vi "waveform_array_to_xy_array.vi"(1 "waveform array":waveform(dbl)[](array[waveform])) -> (0 "XY array":cluster{timestamp[], "Y":dbl[]}[](array[cluster]))   [LabVIEW 2019]
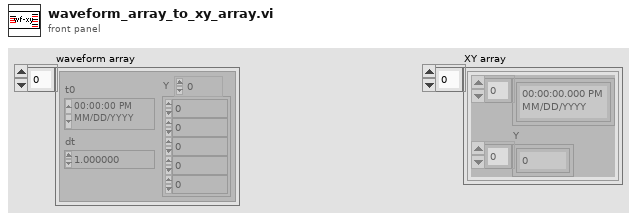
[diagram p1: front panel]
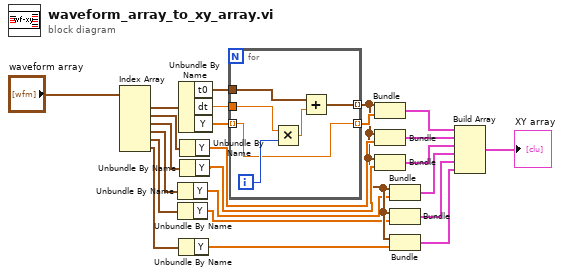
[diagram p0: block diagram]
diagram:
  n1 = Index Array(array="waveform array") -> (element #1=w23:waveform(dbl), element #2=w19:waveform(dbl), element #3=w16:waveform(dbl), element #4=w10:waveform(dbl), element #5=w9:waveform(dbl), element #6=w8:waveform(dbl))  [unwired: 6 in]
  n2 = Unbundle By Name(w10) -> ("Y"=w6:dbl[])
  n3 = Unbundle By Name(w9) -> ("Y"=w5:dbl[])
  n4 = Unbundle By Name(w23) -> ("t0"=w22:timestamp, "dt"=w24:dbl, "Y"=w21:dbl[])
  n5 = Unbundle By Name(w8) -> ("Y"=w4:dbl[])
  n6 = Unbundle By Name(w19) -> ("Y"=w18:dbl[])
  n7 = Unbundle By Name(w16) -> ("Y"=w17:dbl[])
  n8 = for {
    tunnel: w24 -> [w30]
    tunnel: w22 -> [w27]
    tunnel: w21 -> [w26] mode=indexing
    tunnel: [w26] -> w20 mode=indexing
    tunnel: [w25] -> w7 mode=indexing
    i -> [w28]
    n9 = Multiply(x=w30, y=w28) -> (x*y=w29:dbl)
    n10 = Add(x=w27, y=w29) -> (x+y=w25:timestamp)
  }
  n11 = Bundle(w7, w20) -> (w14:cluster{timestamp[], dbl[]})  [unwired: 1 in]
  n12 = Bundle(w7, "Y"=w18) -> (w13:cluster{timestamp[], "Y":dbl[]})  [unwired: 1 in]
  n13 = Bundle(w7, "Y"=w17) -> (w12:cluster{timestamp[], "Y":dbl[]})  [unwired: 1 in]
  n14 = Bundle(w7, "Y"=w6) -> (w3:cluster{timestamp[], "Y":dbl[]})  [unwired: 1 in]
  n15 = Bundle(w7, "Y"=w5) -> (w2:cluster{timestamp[], "Y":dbl[]})  [unwired: 1 in]
  n16 = Bundle(w7, "Y"=w4) -> (w1:cluster{timestamp[], "Y":dbl[]})  [unwired: 1 in]
  n17 = Build Array(w14, w13, w12, w3, w2, w1) -> (→"XY array":cluster{timestamp[], "Y":dbl[]}[])
